vi "GoToTarget.vi"(0 "object in":refnum<class "5RobotsSkill.lvclass">, 2 "Robot":refnum<class "Robot.lvclass">, 4 "Game":refnum<class "Game.lvclass">, 5 "error in (no error)":errorcluster) -> (14 "object out":refnum<class "5RobotsSkill.lvclass">, 16 "reference out":refnum<class "Robot.lvclass">, 19 "error out":errorcluster)   [LabVIEW 2024, in "5RobotsSkill.lvclass"]
uses:
  5RobotsSkill.lvclass
  Robot_class/Robot.lvclass
  Game_class/Game.lvclass
  Robot_class/Robot.lvclass/Robot.ctl
  Game_class/Game.lvclass/Game.ctl
  Game_class/Read BallRef.vi
  Robot_class/Read Zone.vi
  Robot_class/Write dest_orientation.vi
  Robot_class/Write dest_x.vi
  Robot_class/Write dest_y.vi
  Ball_class/Ball.lvclass
  Zone_class/Zone.lvclass
  Utilities_class/Utilities.lvclass
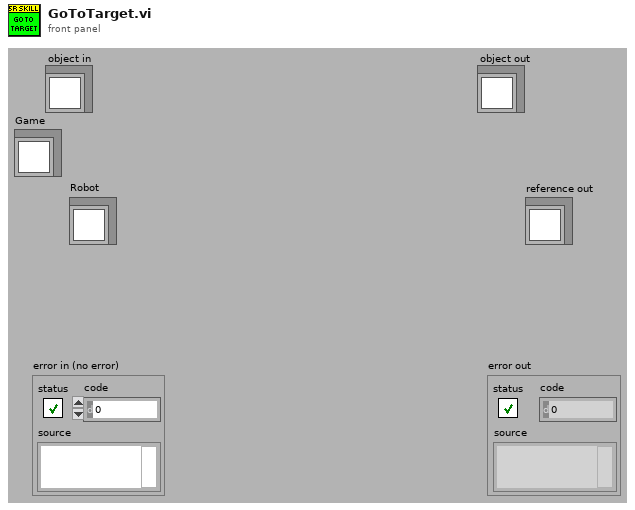
[diagram p1: front panel]
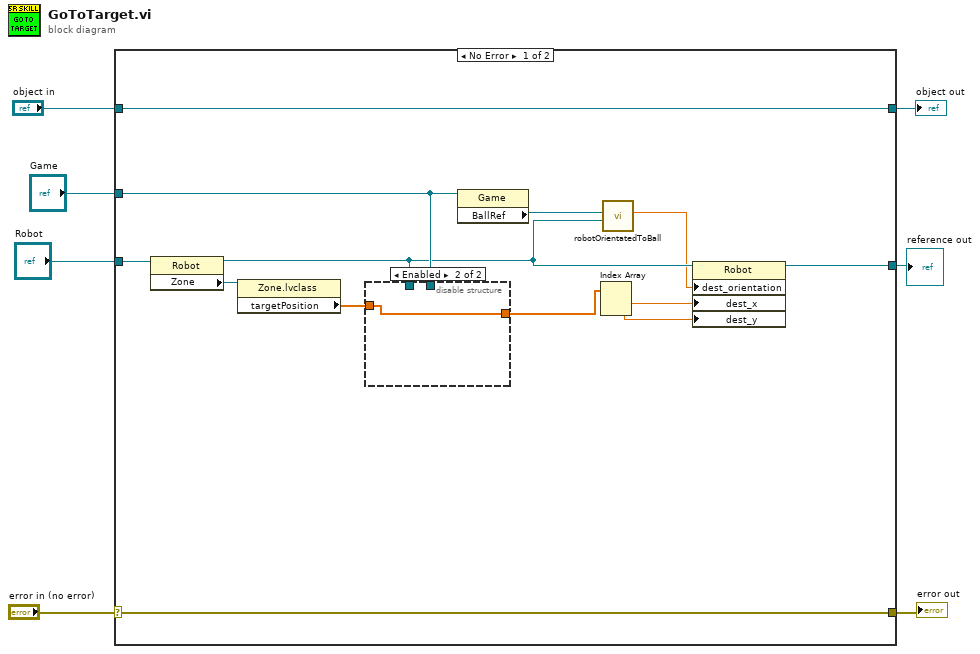
[diagram p0: block diagram]
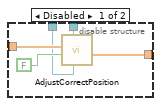
[diagram p2: hidden frame]
diagram:
  n1 = case shown="No Error" "error in (no error)" {
    selector: "error in (no error)" -> [w19 w29]
    tunnel: [w19 w29] -> w6
    tunnel: [w20 w28] -> w4
    tunnel: "object in" -> [w20 w28]
    tunnel: "Robot" -> [w18 w27]
    tunnel: "Game" -> [w15 _]
    tunnel: [w8 w27] -> w1
    frame No Error {
      n2 = property class="Robot"(reference=w18) -> (reference out=w13:refnum<class "Robot.lvclass">, "Zone"=w17:refnum<class "Zone.lvclass">)  [unwired: 1 in, 1 out]
      n3 = property class="Zone.lvclass"(reference=w17) -> ("targetPosition"=w16:dbl[])  [unwired: 1 in, 2 out]
      n4 = disable-structure shown="Enabled" {
        disable-tunnel: w16 -> [w25 w26]
        disable-tunnel: w15 -> [w23 _]
        disable-tunnel: w13 -> [w22 _]
        disable-tunnel: [w21 w26] -> w9
        frame Disabled {
          n5 = call "AdjustCorrectPosition.vi"("Robot"=w22, "Game"=w23, "IsShoot?"=FALSE, "Position"=w25) -> ("AdjustPosition"=w21:dbl[])  [unwired: 5 in, 2 out]
        }
        frame Enabled {
        }
      }
      n6 = property class="Game"(reference=w15) -> ("BallRef"=w14:refnum<class "Ball.lvclass">)  [unwired: 1 in, 2 out]
      n7 = Index Array(array=w9) -> (element #1=w11:dbl, element #2=w10:dbl)  [unwired: 2 in]
      n8 = call "robotOrientatedToBall.vi"("Robot"=w13, "BallRef"=w14) -> ("Orientation"=w12:dbl)  [unwired: 7 in, 2 out]
      n9 = property class="Robot"(reference=w13, "dest_orientation"=w12, "dest_x"=w11, "dest_y"=w10) -> (reference out=w8:refnum<class "Robot.lvclass">)  [unwired: 1 in, 1 out]
    }
    frame Error {
    }
  }
  "error out" <- w6
  "object out" <- w4
  "reference out" <- w1
